vi "Run Video Displays_ABB.vi"   [LabVIEW 2017]
uses:
  ABB global.vi
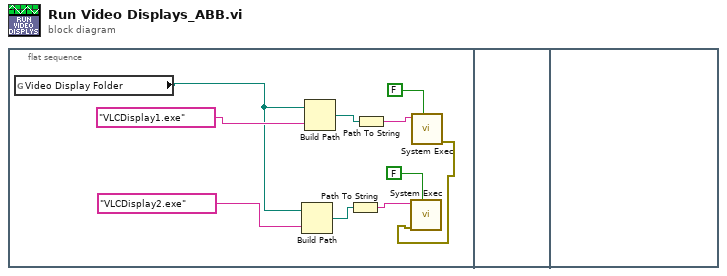
[diagram p0: block diagram]
diagram:
  n1 = flat-sequence {
    frame #0 {
      n2 = global read "ABB global.vi" "Video Display Folder"() -> (w1:path)
      n3 = Build Path(base path=w1, name or relative path="VLCDisplay2.exe") -> (appended path=w4:path)
      n4 = Build Path(base path=w1, name or relative path="VLCDisplay1.exe") -> (appended path=w6:path)
      n5 = Path To String(path=w4) -> (string=w3:string)
      n6 = Path To String(path=w6) -> (string=w5:string)
      n7 = call <vilib>:"System Exec.vi"("wait until completion? (T)"=FALSE, "command line"=w5) -> ("error out"=w2:errorcluster)  [unwired: 6 in, 3 out]
      n8 = call <vilib>:"System Exec.vi"("wait until completion? (T)"=FALSE, "error in (no error)"=w2, "command line"=w3) -> ()  [unwired: 5 in, 4 out]
    }
    frame #1 {
    }
    frame #2 {
    }
  }
